vi "Crosses.vi"() -> ()   [LabVIEW 2014]
uses:
  <vilib>/Utility/file.llb/Read From Spreadsheet File (DBL).vi
  <vilib>/picture/3D Picture Control/NI_3D Picture Control.lvlib
  <vilib>/picture/3D Picture Control/Object/Create Object (name).vi
  Slicer_11-28/LVslicer/Slice/TypeDefs/Area PWRMap Params.ctl
  Slicer_11-28/LVslicer/Slice/TypeDefs/RectHatch.ctl
  Slicer_11-28/LVslicer/Slice/TypeDefs/PowerSpeed.ctl
panel:
  out "Array":T1[](array[typedef])
  out "Layer":dbl
  in  "stop":bool
  out "3D Picture":refnum<vi>(3d-picture)
  out "Crosses":T2(array[cluster])=[{-30.0, 30.0, 382.0, 300.0, 114.6, 229.2, 229.2, 382.0, 382.0}, {-15.0, 30.0, 382.0, 300.0, 95.5, 191.0, 286.5, 382.0, 382.0}, {0.0, 30.0, 327.0, 150.0, 98.1, 196.2, 196.2, 327.0, 327.0}, {15.0, 30.0, 382.0, 300.0, 114.6, 229.2, 229.2, 382.0, 382.0}, {30.0, 30.0, 382.0, 300.0, 152.8, 191.0, 229.2, 267.4, 382.0}, {-30.0, 15.0, 382.0, 300.0, 95.5, 191.0, 286.5, 382.0, 382.0}, {-15.0, 15.0, 327.0, 150.0, 81.75, 163.5, 245.25, 327.0, 327.0}, {0.0, 15.0, 382.0, 300.0, 152.8, 191.0, 229.2, 267.4, 382.0}, {15.0, 15.0, 327.0, 150.0, 130.8, 163.5, 196.2, 228.9, 327.0}, {30.0, 15.0, 382.0, 300.0, 114.6, 229.2, 229.2, 382.0, 382.0}, {-30.0, 0.0, 327.0, 150.0, 98.1, 196.2, 196.2, 327.0, 327.0}, {-15.0, 0.0, 382.0, 300.0, 95.5, 191.0, 286.5, 382.0, 382.0}, {0.0, 0.0, 327.0, 150.0, 81.75, 163.5, 245.25, 327.0, 327.0}, {15.0, 0.0, 382.0, 300.0, 152.8, 191.0, 229.2, 267.4, 382.0}, {30.0, 0.0, 327.0, 150.0, 130.8, 163.5, 196.2, 228.9, 327.0}, {-30.0, -15.0, 382.0, 300.0, 114.6, 229.2, 229.2, 382.0, 382.0}, {-15.0, -15.0, 327.0, 150.0, 98.1, 196.2, 196.2, 327.0, 327.0}, {0.0, -15.0, 382.0, 300.0, 95.5, 191.0, 286.5, 382.0, 382.0}, {15.0, -15.0, 327.0, 150.0, 81.75, 163.5, 245.25, 327.0, 327.0}, {30.0, -15.0, 382.0, 300.0, 152.8, 191.0, 229.2, 267.4, 382.0}, {-30.0, -30.0, 382.0, 300.0, 114.6, 229.2, 229.2, 382.0, 382.0}, {-15.0, -30.0, 382.0, 300.0, 95.5, 191.0, 286.5, 382.0, 382.0}, {0.0, -30.0, 327.0, 150.0, 130.8, 163.5, 196.2, 228.9, 327.0}, {15.0, -30.0, 382.0, 300.0, 152.8, 191.0, 229.2, 267.4, 382.0}, {30.0, -30.0, 327.0, 150.0, 98.1, 196.2, 196.2, 327.0, 327.0}]
  in  "Save?":bool
  in  "Path":path=path "C:/Users/deane1/Documents/GitHub/TestRuns"
  in  "HighPower":dbl=500.0
  in  "Display":T3={"Mode"=enum."Inherit Value", "PointSize"=1.0, "LineWidth"=1.0}
  in  "LayerEnd":u32=170
  in  "LayerStart":u32=170
  in  "HatchPow":T4={"Power"=300.0, "Mark Speed"=400.0, "Jump Speed"=1000.0}
  in  "RectHatch":T5={"Width"=10.0, "Height"=10.0, "Angle"=45.0, "OffX"=0.1, "OffY"=0.1, "Spacing"=0.1} {"Spacing" format="%#_13g"; "OffY" format="%#_13g"; "OffX" format="%#_13g"; "Height" format="%#_13g"; "Width" format="%#_13g"}
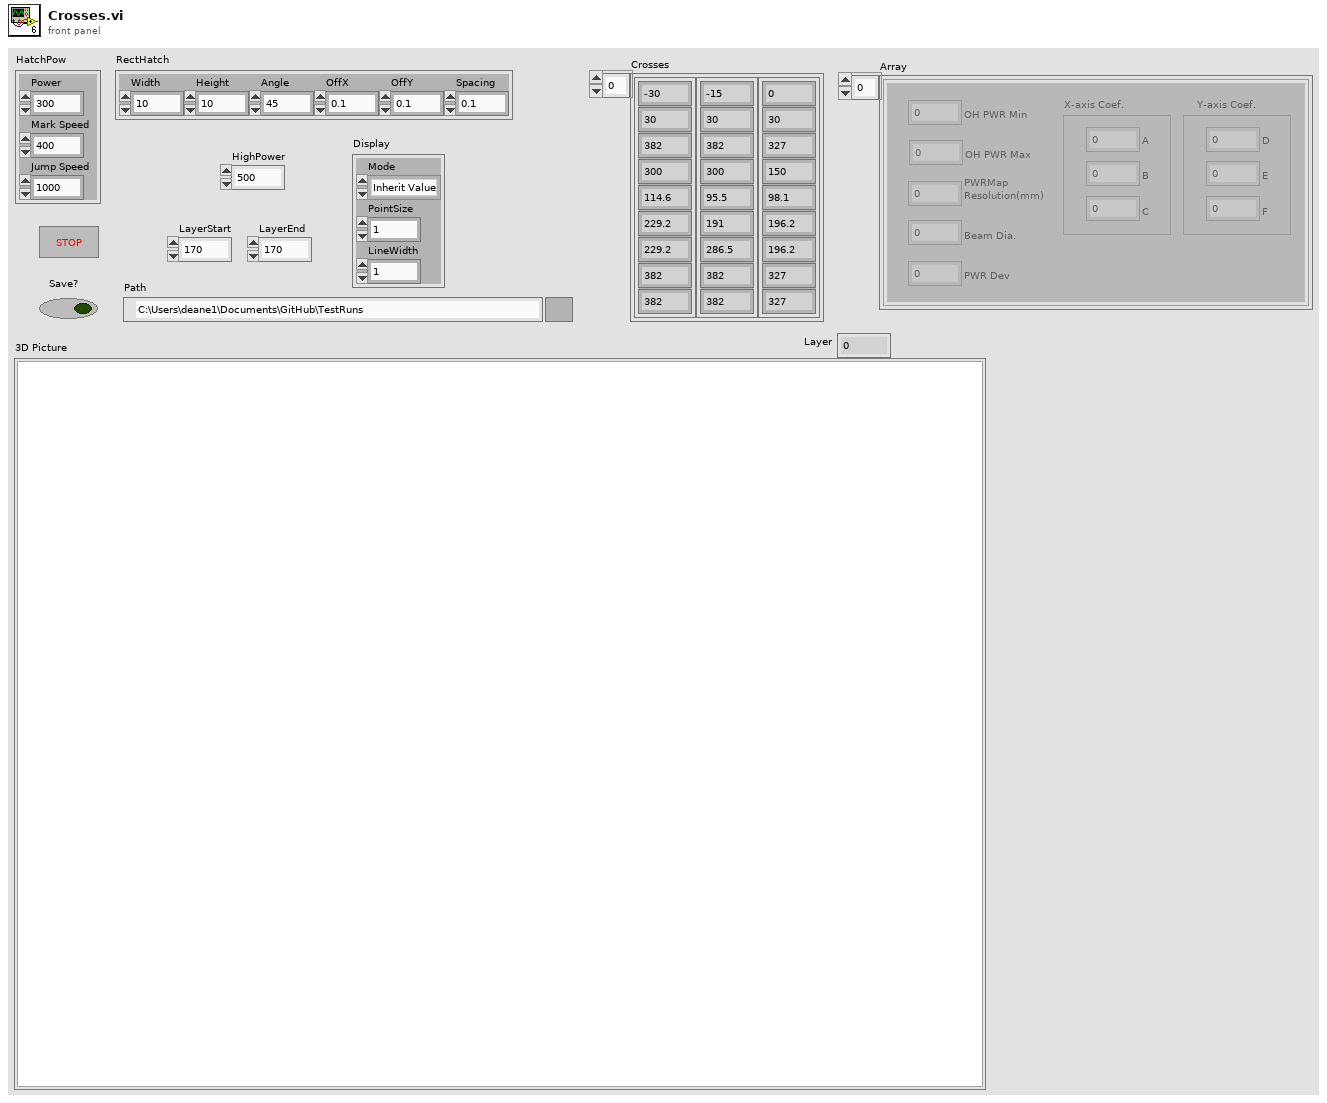
[diagram p1: front panel]
types:
  T1 = typedef "Area PWRMap Params.ctl" = cluster{"PWRMap \nResolution(mm)":dbl, "Beam Dia.":sgl, "PWR Dev":u32, "OH PWR Min":dbl, "X-axis Coef.":cluster{"A":dbl, "B":dbl, "C":dbl}, "OH PWR Max":dbl, "Y-axis Coef.":cluster{"D":dbl, "E":dbl, "F":dbl}}
  T2 = cluster{dbl, dbl, dbl, dbl, dbl, dbl, dbl, dbl, dbl}[]
  T3 = cluster{"Mode":enum16{"Inherit Value", "Points", "Wireframe", "Polygons"}, "PointSize":sgl, "LineWidth":sgl}
  T4 = typedef "PowerSpeed.ctl" = cluster{"Power":dbl, "Mark Speed":dbl, "Jump Speed":dbl}
  T5 = typedef "RectHatch.ctl" = cluster{"Width":dbl, "Height":dbl, "Angle":sgl, "OffX":dbl, "OffY":dbl, "Spacing":dbl}
  T6 = cluster{dbl, dbl, dbl, dbl, dbl, dbl, dbl, dbl, dbl}
  T7 = typedef "PathSupreme.ctl" = cluster{"VelocityProfiles":T8[], "Path":T9}
  T8 = typedef "VelocityProfile.ctl" = cluster{"ID":u32, "Velocity":dbl, "Mode":string, "tV1":u32, "tV2":u32, "tL1":u32, "tL2":u32}
  T9 = typedef "PathCut.ctl" = cluster{"Type":string, "Tag":string, "Segments":T10[]}
  T10 = typedef "Segment.ctl" = cluster{"SegmentID":u16, "Power":sgl, "idxVelocityProfile":u16, "End":cluster{"X":sgl, "Y":sgl}}
  T11 = typedef "Point3D.ctl" = cluster{"X":sgl, "Y":sgl, "Z":sgl}
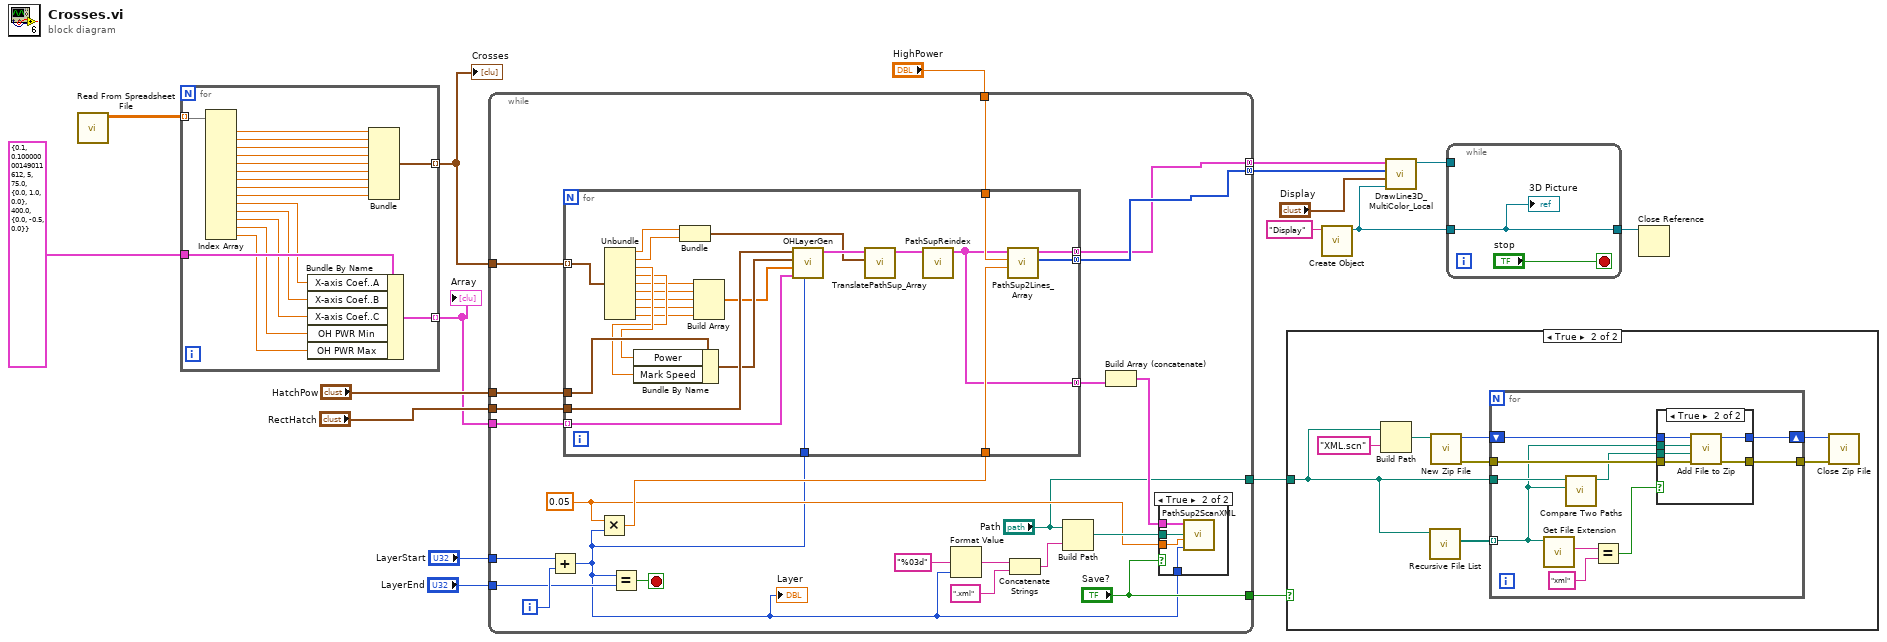
[diagram p0: block diagram]
diagram:
  n1 = call-poly <vilib>:"Read From Spreadsheet File.vi"() -> ("all rows"=w18:dbl[][])  [unwired: 7 in, 4 out]
  n2 = for {
    tunnel: w18 -> [w36] mode=indexing
    tunnel: [w31] -> w16 mode=indexing
    tunnel: T1 {"PWRMap \nResolution(mm)"=0.1, "Beam Dia."=0.1, "PWR Dev"=5, "OH PWR Min"=75.0, "X-axis Coef."={"A"=0.0, "B"=1.0, "C"=0.0}, "OH PWR Max"=400.0, "Y-axis Coef."={"D"=0.0, "E"=-0.5, "F"=0.0}} ("OH Power Map  Params (mm, Watts)") -> [w25]
    tunnel: [w21] -> w11 mode=indexing
    n3 = Index Array(array=w36) -> (element #1=w34:dbl, element #2=w35:dbl, element #3=w33:dbl, element #4=w32:dbl, element #5=w30:dbl, element #6=w29:dbl, element #7=w28:dbl, element #8=w27:dbl, element #9=w26:dbl, element #10=w22:dbl, element #11=w23:dbl, element #12=w24:dbl, element #13=w20:dbl, element #14=w19:dbl)  [unwired: 14 in]
    n4 = Bundle By Name(cluster=w25, "X-axis Coef..A"=w22, "X-axis Coef..B"=w23, "X-axis Coef..C"=w24, "OH PWR Min"=w20, "OH PWR Max"=w19) -> (w21:T1)
    n5 = Bundle(w34, w35, w33, w32, w30, w29, w28, w27, w26) -> (w31:T6)  [unwired: 1 in]
  }
  "Crosses" <- w16
  "Array" <- w11
  n6 = while {
    tunnel: "HighPower" -> [w39]
    tunnel: [w37] -> w10 mode=concatenating
    tunnel: [w38] -> w9 mode=concatenating
    tunnel: w16 -> [w57]
    tunnel: "RectHatch" -> [w47]
    tunnel: "HatchPow" -> [w46]
    tunnel: "LayerEnd" -> [w56]
    tunnel: "LayerStart" -> [w55]
    tunnel: w11 -> [w45]
    tunnel: ["Path"] -> w4
    tunnel: ["Save?"] -> w2
    i -> [w59]
    stop <- w58 stop-if-true
    w43 = 0.05 ("y")
    n7 = Add(x=w55, y=w59) -> (x+y=w40:u32)
    "Layer" <- w40
    n8 = Multiply(x=w43, y=w40) -> (x*y=w49:dbl)
    n9 = for {
      tunnel: w40 -> [w87]
      tunnel: w49 -> [w81]
      tunnel: w39 -> [w78]
      tunnel: [w86] -> w37 mode=concatenating
      tunnel: w57 -> [w85] mode=indexing
      tunnel: w47 -> [w84]
      tunnel: w46 -> [w76]
      tunnel: [w64] -> w48 mode=concatenating
      tunnel: [w77] -> w38 mode=concatenating
      tunnel: w45 -> [w66] mode=indexing
      n10 = Unbundle(w85) -> (w83:dbl, w82:dbl, w74:dbl, w73:dbl, w72:dbl, w71:dbl, w70:dbl, w69:dbl, w68:dbl)
      n11 = Bundle By Name(cluster=w76, "Power"=w74, "Mark Speed"=w73) -> (w75:T4)
      n12 = Bundle(w83, w82) -> (w79:cluster{dbl, dbl})  [unwired: 1 in]
      n13 = Build Array(w72, w71, w70, w69, w68) -> (w67:dbl[])
      n14 = call "OHLayerGen.vi"("Layer"=w87, "OH Power Map \nParams (mm, Watts)"=w66, "OHpows"=w67, "HatchPow"=w75, "RectHatch"=w84) -> ("PathSups"=w80:T7[])  [unwired: 6 in]
      n15 = call "TranslatePathSup_Array.vi"("Offset"=w79, "PathSupsIn"=w80) -> ("PathSupsOut"=w65:T7[])  [unwired: 9 in]
      n16 = call "PathSupReindex.vi"("PathSupremes"=w65) -> ("PathSupOut"=w64:T7[])  [unwired: 10 in]
      n17 = call "PathSup2Lines_Array.vi"("Z"=w81, "HighPower"=w78, "PathSupIn"=w64) -> ("Colors"=w77:u32[], "Lines"=w86:cluster{"P0":T11, "P1":T11}[])  [unwired: 7 in]
    }
    n18 = Equal?(x=w40, y=w56) -> (x = y?=w58:bool)
    n19 = Format Value(format string="%03d", value (0)=w40) -> (output string=w53:string)  [unwired: 1 in]
    n20 = Concatenate Strings(w53, ".xml" ("string")) -> (w51:string)
    n21 = Build Path(base path="Path", name or relative path=w51) -> (appended path=w50:path)
    n22 = Build Array (concatenate)(w48) -> (w44:T7[])  [unwired: 1 in]
    n23 = case shown="True" "Save?" {
      tunnel: w44 -> [_ w63]
      tunnel: w50 -> [_ w62]
      tunnel: w43 -> [_ w61]
      tunnel: w40 -> [_ w60]
      frame False {
      }
      frame True {
        n24 = call "PathSup2ScanXML.vi"("PathSupremes"=w63, "Path"=w62, "Thickness"=w61, "layer"=w60) -> ()  [unwired: 4 in, 1 out]
      }
    }
  }
  n25 = case shown="True" w2 {
    tunnel: w4 -> [_ w95]
    frame False {
    }
    frame True {
      n26 = Build Path(base path=w95, name or relative path="XML.scn") -> (appended path=w88:path)
      n27 = call <vilib>:"Recursive File List.vi"("Folder Path"=w95) -> ("All Files in Dir"=w90:path[])  [unwired: 6 in, 4 out]
      n28 = call <vilib>:"New Zip File.vi"("target"=w88) -> ("error out"=w94:errorcluster, "zip file out"=w93:i64)  [unwired: 4 in, 1 out]
      n29 = for {
        shift-right: [w102] -> w91
        shift-left: w93 -> [w104]
        tunnel: w94 -> [w105]
        tunnel: [w103] -> w92
        tunnel: w90 -> [w97] mode=indexing
        tunnel: w95 -> [w98]
        n30 = call <vilib>:"Get File Extension.vi"("file"=w97) -> ("lowercase file extension"=w101:string)  [unwired: 7 in, 3 out]
        n31 = call <vilib>:"Compare Two Paths.vi"("Path 2"=w97, "Path 1"=w98) -> ("Relative Path from 1 to 2"=w96:path)  [unwired: 6 in, 3 out]
        n32 = Equal?(x=w101, y="xml") -> (x = y?=w99:bool)
        n33 = case shown="True" w99 {
          tunnel: w105 -> [w106 w113]
          tunnel: w104 -> [w107 w112]
          tunnel: [w106 w111] -> w103
          tunnel: [w107 w110] -> w102
          tunnel: w97 -> [_ w109]
          tunnel: w96 -> [_ w108]
          frame False {
          }
          frame True {
            n34 = call <vilib>:"Add File to Zip.vi"("error in (no error)"=w113, "destination path in zip"=w108, "source file path"=w109, "zip file in"=w112) -> ("error out"=w111:errorcluster, "zip file out"=w110:i64)  [unwired: 6 in]
          }
        }
      }
      n35 = call <vilib>:"Close Zip File.vi"("error in (no error)"=w92, "zip file in"=w91) -> ()  [unwired: 5 in, 1 out]
    }
  }
  n36 = call-poly <vilib>:"Create Object.vi"("Name"="Display") -> ("Scene:New Object"=w5:refnum<vi>)  [unwired: 9 in, 1 out]
  n37 = call "DrawLine3D_MultiColor_Local.vi"("Scene Object In"=w5, "Display"="Display", "Colors"=w9, "Lines"=w10) -> ("Scene Object Out"=w1:refnum<vi>)  [unwired: 7 in]
  n38 = while {
    tunnel: w5 -> [w115]
    tunnel: [w115] -> w6
    tunnel: w1 -> [_]
    stop <- "stop" stop-if-true
    "3D Picture" <- w115
  }
  n39 = Close Reference(reference=w6) -> ()  [unwired: 1 in, 1 out]
